vi "Read K_D.vi"(8 "error in (no error)":errorcluster, 11 "PID Controller in":refnum<class "PID Controller.lvclass">) -> (0 "error out":errorcluster, 2 "K_D":T1, 3 "PID Controller out":refnum<class "PID Controller.lvclass">)   [LabVIEW 2014, in "Controller Library.lvlib" / "PID Controller.lvclass"]
uses:
  PID Controller.lvclass
  <vilib>/Analysis/Matrix/Datatypes/RealMatrix.ctl
  PID Controller.lvclass/PID Controller.ctl
  <vilib>/Analysis/Matrix/NI_Matrix.lvlib
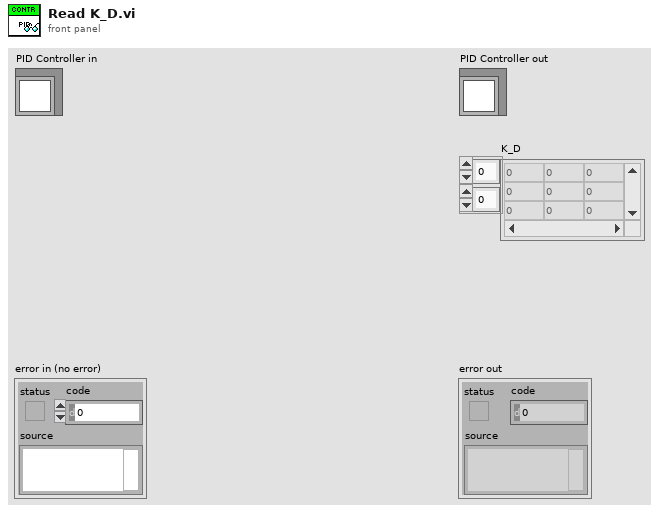
[diagram p1: front panel]
types:
  T1 = typedef "NI_Matrix.lvlib/RealMatrix.ctl" = dbl[][]
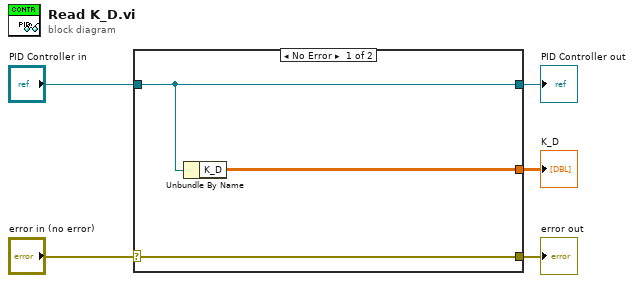
[diagram p0: block diagram]
diagram:
  n1 = case shown="No Error" "error in (no error)" {
    selector: "error in (no error)" -> [w8 w9]
    tunnel: [w8 w9] -> w4
    tunnel: [w7 w10] -> w2
    tunnel: "PID Controller in" -> [w7 w10]
    tunnel: [w6 _] -> w1
    frame No Error {
      n2 = Unbundle By Name(w7) -> ("K_D"=w6:T1)
    }
    frame Error {
    }
  }
  "error out" <- w4
  "PID Controller out" <- w2
  "K_D" <- w1
